vi "Front Right Wheel.vi"(9 "output cluster 2":T2, 10 "Pot Val in":dbl, 11 "Wheel Angle Offset":dbl) -> (0 "Wheel Angle":dbl, 1 "Drive Speed":dbl, 3 "Wheel Speed":dbl)   [LabVIEW 2019]
uses:
  <vilib>/addons/control/pid/pid.llb/PID (DBL).vi
  <vilib>/addons/control/pid/NI_PID_pid.lvlib
panel:
  in  "PID gains":T1={"proportional gain (Kc)"=0.01, "integral time (Ti, min)"=0.0, "derivative time (Td, min)"=0.0} {"derivative time (Td, min)" format="%.3f"; "integral time (Ti, min)" format="%.3f"; "proportional gain (Kc)" format="%.3f"}
  out "Requested Angle":dbl
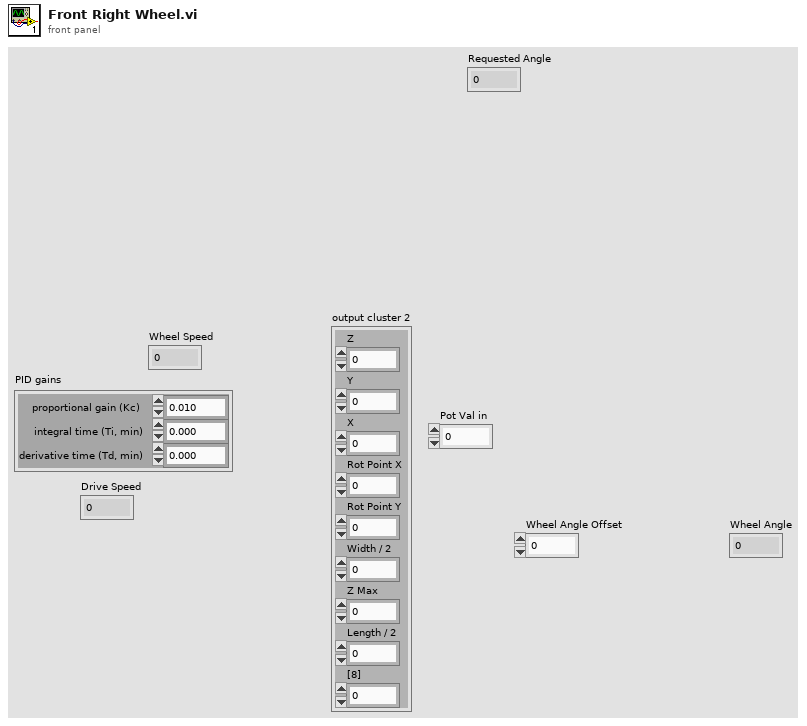
[diagram p1: front panel]
types:
  T1 = cluster{"proportional gain (Kc)":dbl, "integral time (Ti, min)":dbl, "derivative time (Td, min)":dbl}
  T2 = cluster{"Z":dbl, "Y":dbl, "X":dbl, "Rot Point X":dbl, "Rot Point Y":dbl, "Width / 2":dbl, "Z Max":dbl, "Length / 2":dbl, "[8]":dbl}
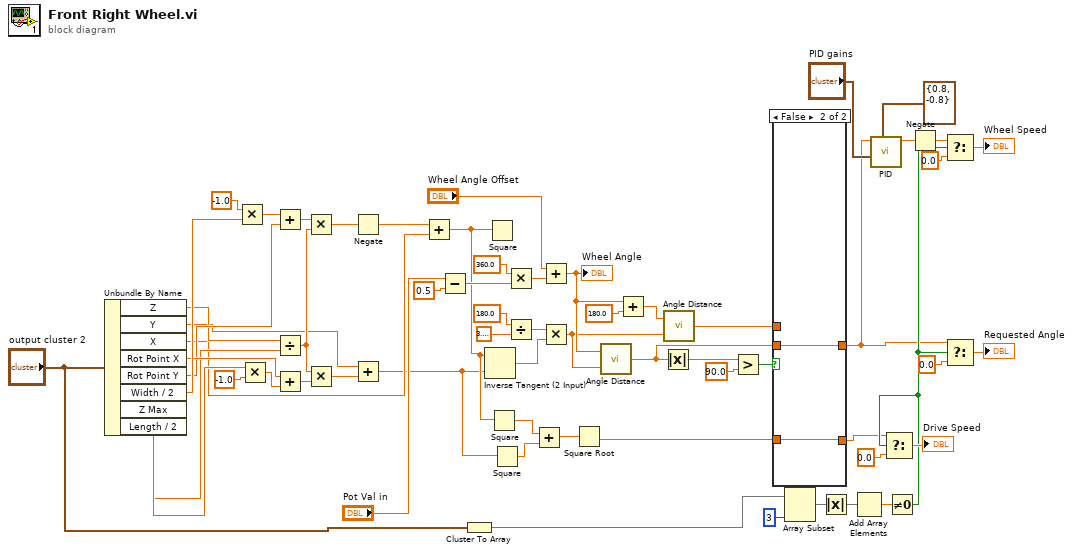
[diagram p0: block diagram]
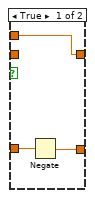
[diagram p2: hidden frame]
diagram:
  n1 = Unbundle By Name("output cluster 2") -> ("Z"=w29:dbl, "Y"=w27:dbl, "X"=w26:dbl, "Rot Point X"=w31:dbl, "Rot Point Y"=w30:dbl, "Width / 2"=w59:dbl, "Z Max"=w28:dbl, "Length / 2"=w60:dbl)
  n2 = Multiply(x=-1.0, y=w59) -> (x*y=w39:dbl)
  n3 = Multiply(x=w60, y=-1.0) -> (x*y=w38:dbl)
  n4 = Add(x=w39, y=w30) -> (x+y=w40:dbl)
  n5 = Divide(x=w29, y=w28) -> (x/y=w44:dbl)
  n6 = Add(x=w31, y=w38) -> (x+y=w45:dbl)
  n7 = Multiply(x=w40, y=w44) -> (x*y=w42:dbl)
  n8 = Multiply(x=w44, y=w45) -> (x*y=w43:dbl)
  n9 = Negate(x=w42) -> (-x=w41:dbl)
  n10 = Add(x=w27, y=w43) -> (x+y=w4:dbl)
  n11 = Add(x=w41, y=w26) -> (x+y=w5:dbl)
  n12 = Subtract(x="Pot Val in", y=0.5) -> (x-y=w57:dbl)
  n13 = Cluster To Array(cluster="output cluster 2") -> (array=w18:dbl[])
  n14 = Inverse Tangent (2 Input)(1:w4, 2:w5) -> (0:w49:dbl)
  n15 = Square(x=w5) -> ()  [unwired: 1 out]
  n16 = Square(x=w5) -> (x^2=w12:dbl)
  n17 = Square(x=w4) -> (x^2=w11:dbl)
  n18 = Multiply(x=360.0 ("y"), y=w57) -> (x*y=w55:dbl)
  n19 = Divide(x=180.0 ("y"), y=3.141592653589793) -> (x/y=w48:dbl)
  n20 = Add(x=w12, y=w11) -> (x+y=w13:dbl)
  n21 = Add(x="Wheel Angle Offset", y=w55) -> (x+y=w50:dbl)
  "Wheel Angle" <- w50
  n22 = Multiply(x=w48, y=w49) -> (x*y=w37:dbl)
  n23 = Square Root(x=w13) -> (sqrt(x)=w6:dbl)
  n24 = call "Angle Distance.vi"("target angle"=w37, "current angle"=w50) -> ("distance"=w32:dbl)
  n25 = Add(x=w50, y=180.0) -> (x+y=w51:dbl)
  n26 = Absolute Value(x=w32) -> (abs(x)=w35:dbl)
  n27 = call "Angle Distance.vi"("target angle"=w37, "current angle"=w51) -> ("distance"=w33:dbl)
  n28 = Greater?(x=w35, y=90.0) -> (0:w34:bool)
  n29 = case shown="False" w34 {
    tunnel: w33 -> [w65 _]
    tunnel: w32 -> [_ w67]
    tunnel: [w65 w67] -> w3
    tunnel: [w64 w66] -> w7
    tunnel: w6 -> [w63 w66]
    frame True {
      n30 = Negate(x=w63) -> (-x=w64:dbl)
    }
    frame False {
    }
  }
  n31 = Array Subset(array=w18, length=3) -> (w24:dbl[])  [unwired: 1 in]
  n32 = Absolute Value(x=w24) -> (abs(x)=w21:dbl[])
  n33 = Add Array Elements(numeric array=w21) -> (sum=w25:dbl)
  n34 = call-poly <vilib>:"PID.vi"("output range"=cluster{"output high":dbl, "output low":dbl} {"output high"=0.8, "output low"=-0.8}, "PID gains"="PID gains", "setpoint"=w3) -> ("output"=w2:dbl)  [unwired: 7 in, 1 out]
  n35 = Not Equal To 0?(x=w25) -> (x != 0?=w8:bool)
  n36 = Select(t=w7, s=w8, f=0.0) -> (s? t:f=→"Drive Speed":dbl)
  n37 = Negate(x=w2) -> (-x=w1:dbl)
  n38 = Select(t=w1, s=w8, f=0.0) -> (s? t:f=→"Wheel Speed":dbl)
  n39 = Select(t=w3, s=w8, f=0.0) -> (s? t:f=→"Requested Angle":dbl)
